vi "LOG_sim_2 (SubVI).vi"(3 "Data File":dbl[][](array[numeric]), 4 "Rotation":T5, 5 "Time":T3, 6 "TVA":T2, 7 "Position":T4, 9 "output Rocket Dynamics":T1) -> ()   [LabVIEW 2017]
panel:
  out "output array":dbl[](array[numeric])
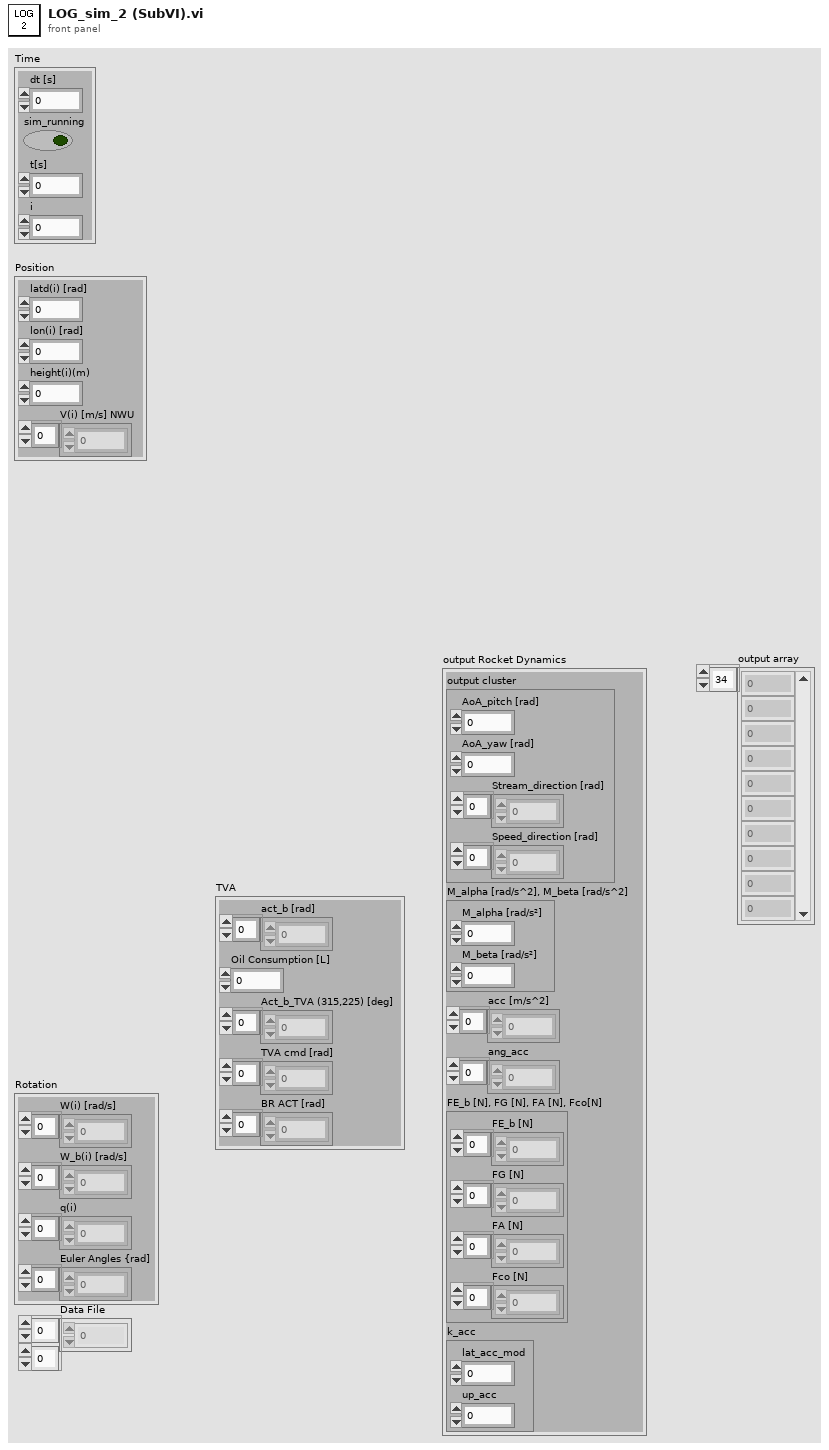
[diagram p1: front panel]
types:
  T1 = cluster{"output cluster":cluster{"AoA_pitch [rad]":dbl, "AoA_yaw [rad]":dbl, "Stream_direction [rad]":dbl[], "Speed_direction [rad]":dbl[]}, "M_alpha [rad/s^2], M_beta [rad/s^2]":cluster{"M_alpha [rad/s²]":dbl, "M_beta [rad/s²]":dbl}, "acc [m/s^2]":dbl[], "ang_acc":dbl[], "FE_b [N], FG [N], FA [N], Fco[N]":cluster{"FE_b [N]":dbl[], "FG [N]":dbl[], "FA [N]":dbl[], "Fco [N]":dbl[]}, "k_acc":cluster{"lat_acc_mod":dbl, "up_acc":dbl}}
  T2 = cluster{"act_b [rad]":dbl[], "Oil Consumption [L]":dbl, "Act_b_TVA (315,225) [deg]":dbl[], "TVA cmd [rad]":dbl[], "BR ACT [rad]":dbl[]}
  T3 = cluster{"dt [s]":dbl, "sim_running":bool, "t[s]":dbl, "i":i32}
  T4 = cluster{"latd(i) [rad]":dbl, "lon(i) [rad]":dbl, "height(i)(m)":dbl, "V(i) [m/s] NWU":dbl[]}
  T5 = cluster{"W(i) [rad/s]":dbl[], "W_b(i) [rad/s]":dbl[], "q(i)":dbl[], "Euler Angles {rad]":dbl[]}
  T6 = cluster{"M_alpha [rad/s²]":dbl, "M_beta [rad/s²]":dbl}
  T7 = cluster{"AoA_pitch [rad]":dbl, "AoA_yaw [rad]":dbl, "Stream_direction [rad]":dbl[], "Speed_direction [rad]":dbl[]}
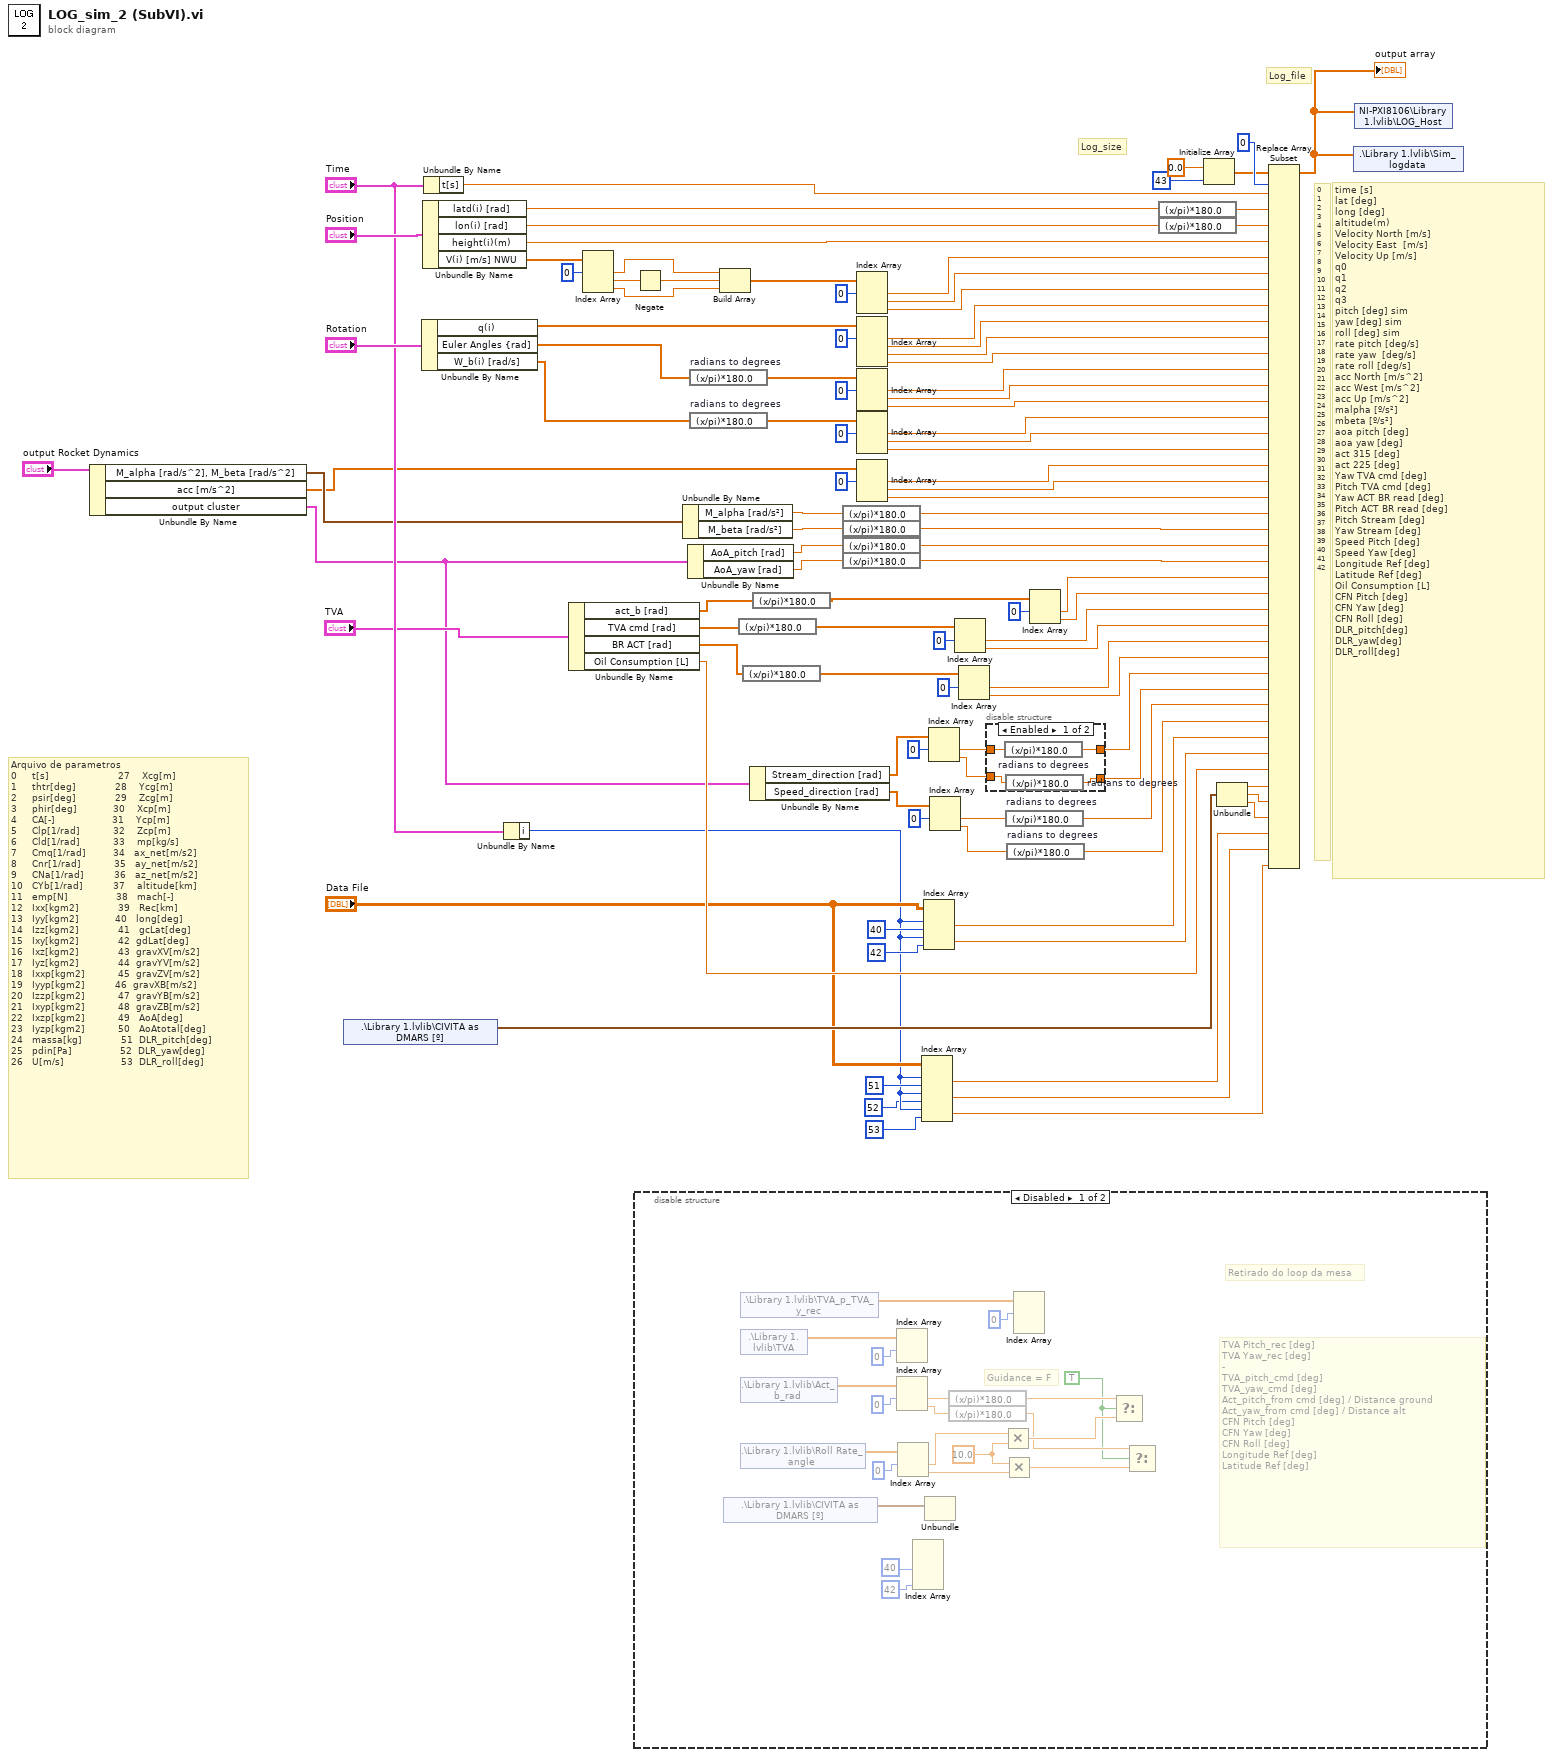
[diagram p0: block diagram]
diagram:
  # "Arquivo de parametros\n0     t[s]                       27    Xcg[m] \n1     thtr[deg]             28    Ycg[m]\n2     psir[deg]             29    Zcg[m]  \n3     phir[deg]            30    Xcp[m]       \n4     CA[-]                   31    Ycp[m]        \n5     Clp[1/rad]           32    Zcp[m]     \n6     Cld[1/rad]           33    mp[kg/s]        \n7     Cmq[1/rad]         34   ax_net[m/s2]         \n8     Cnr[1/rad]           35   ay_net[m/s2]      \n9     CNa[1/rad]          36   az_net[m/s2]      \n10   CYb[1/rad]          37    altitude[km]       \n11   emp[N]                38   mach[-]     \n12   Ixx[kgm2]             39   Rec[km]     \n13   Iyy[kgm2]            40   long[deg]     \n14   Izz[kgm2]             41   gcLat[deg]        \n15   Ixy[kgm2]             42  gdLat[deg]       \n16   Ixz[kgm2]             43  gravXV[m/s2]  \n17   Iyz[kgm2]             44  gravYV[m/s2]     \n18   Ixxp[kgm2]           45  gravZV[m/s2]         \n19   Iyyp[kgm2]          46  gravXB[m/s2]         \n20   Izzp[kgm2]           47  gravYB[m/s2]         \n21   Ixyp[kgm2]           48  gravZB[m/s2]           \n22   Ixzp[kgm2]           49   AoA[deg]             \n23   Iyzp[kgm2]           50   AoAtotal[deg]       \n24   massa[kg]             51  DLR_pitch[deg]    \n25   pdin[Pa]                52  DLR_yaw[deg]  \n26   U[m/s]                   53  DLR_roll[deg]"
  # "Log_file"
  # "Log_size"
  # "0\n1\n2\n3\n4\n5\n6\n7\n8\n9\n10\n11\n12\n13\n14\n15\n16\n17\n18\n19\n20\n21\n22\n23\n24\n25\n26\n27\n28\n29\n30\n31\n32\n33 34 35\n36373839\n40\n41\n42"
  # "time [s]\nlat [deg]\nlong [deg]\naltitude(m)\nVelocity North [m/s]\nVelocity East  [m/s]\nVelocity Up [m/s]\nq0\nq1\nq2\nq3\npitch [deg] sim\nyaw [deg] sim\nroll [deg] sim\nrate pitch [deg/s] \nrate yaw  [deg/s]\nrate roll [deg/s]\nacc North [m/s^2] \nacc West [m/s^2]\nacc Up [m/s^2]\nmalpha [º/s²]\nmbeta [º/s²]\naoa pitch [deg] \naoa yaw [deg]\nact 315 [deg] \nact 225 [deg]\nYaw TVA cmd [deg]\nPitch TVA cmd [deg]\nYaw ACT BR read [deg]\nPitch ACT BR read [deg]\nPitch Stream [deg]\nYaw Stream [deg]\nSpeed Pitch [deg]\nSpeed Yaw [deg]\nLongitude Ref [deg]\nLatitude Ref [deg]\nOil Consumption [L]\nCFN Pitch [deg]\nCFN Yaw [deg]\nCFN Roll [deg]\nDLR_pitch[deg]  \nDLR_yaw[deg] \nDLR_roll[deg]"
  n1 = Unbundle By Name("output Rocket Dynamics") -> ("M_alpha [rad/s^2], M_beta [rad/s^2]"=w11:T6, "acc [m/s^2]"=w10:dbl[], "output cluster"=w9:T7)
  n2 = shared-variable ".\\Library 1.lvlib\\CIVITA as DMARS [º]"() -> (w16:cluster{"phi":dbl, "theta":dbl, "psi":dbl})  [unwired: 1 in, 1 out]
  n3 = Unbundle By Name("Rotation") -> ("q(i)"=w103:dbl[], "Euler Angles {rad]"=w37:dbl[], "W_b(i) [rad/s]"=w36:dbl[])
  n4 = Unbundle By Name("Position") -> ("latd(i) [rad]"=w98:dbl, "lon(i) [rad]"=w99:dbl, "height(i)(m)"=w100:dbl, "V(i) [m/s] NWU"=w101:dbl[])
  n5 = Unbundle By Name("Time") -> ("t[s]"=w95:dbl)
  n6 = Unbundle By Name("Time") -> ("i"=w6:i32)
  n7 = Unbundle By Name("TVA") -> ("act_b [rad]"=w26:dbl[], "TVA cmd [rad]"=w28:dbl[], "BR ACT [rad]"=w21:dbl[], "Oil Consumption [L]"=w24:dbl)
  n8 = Index Array(array=w101, index #1=0 ("index")) -> (element #1=w73:dbl, element #2=w71:dbl, element #3=w74:dbl)  [unwired: 2 in]
  n9 = Negate(x=w71) -> (-x=w72:dbl)
  n10 = disable-structure shown="Disabled" {
    frame Disabled {
      w114 = TRUE ("s")
      w121 = 10.0 ("x")
      # "TVA Pitch_rec [deg]\nTVA Yaw_rec [deg]\n-\nTVA_pitch_cmd [deg]\nTVA_yaw_cmd [deg]\nAct_pitch_from cmd [deg] / Distance ground\nAct_yaw_from cmd [deg] / Distance alt\nCFN Pitch [deg]\nCFN Yaw [deg]\nCFN Roll [deg]\nLongitude Ref [deg]\nLatitude Ref [deg]"
      # "Retirado do loop da mesa"
      # "Guidance = F"
      n11 = shared-variable ".\\Library 1.lvlib\\CIVITA as DMARS [º]"() -> (w113:cluster{"phi":dbl, "theta":dbl, "psi":dbl})  [unwired: 1 in, 1 out]
      n12 = shared-variable ".\\Library 1.lvlib\\TVA_p_TVA_y_rec"() -> (w130:dbl[])  [unwired: 1 in, 1 out]
      n13 = shared-variable ".\\Library 1.lvlib\\TVA"() -> (w133:dbl[])  [unwired: 1 in, 1 out]
      n14 = shared-variable ".\\Library 1.lvlib\\Act_b_rad"() -> (w128:dbl[])  [unwired: 1 in, 1 out]
      n15 = shared-variable ".\\Library 1.lvlib\\Roll Rate_angle"() -> (w124:dbl[])  [unwired: 1 in, 1 out]
      n16 = Index Array(array=w133, index #1=0 ("index")) -> (element #1=w132:dbl, element #2=w131:dbl)  [unwired: 1 in]
      n17 = Index Array(array=w128, index #1=0 ("index")) -> (element #1=w127:dbl, element #2=w126:dbl)  [unwired: 1 in]
      n18 = Index Array(array=w124, index #1=0 ("index")) -> (element #1=w123:dbl, element #2=w122:dbl)  [unwired: 1 in]
      n19 = Index Array(index (col) #1=40 ("index"), index (row) #2=w108, index (col) #2=42 ("index")) -> (element #1=w106, index (row) #1=w108:i32, element #2=w105)  [unwired: 1 in]
      n20 = Unbundle(w113) -> ("phi"=w112:dbl, "theta"=w111:dbl, "psi"=w110:dbl)
      n21 = expression code="(x/pi)*180.0" ("radians to degrees")(w127) -> (w120:dbl)
      n22 = expression code="(x/pi)*180.0" ("radians to degrees")(w126) -> (w118:dbl)
      n23 = Multiply(x=w123, y=w121) -> (x*y=w119:dbl)
      n24 = Multiply(x=w121, y=w122) -> (x*y=w117:dbl)
      n25 = Index Array(array=w130, index #1=0 ("index")) -> (element #1=w137:dbl, element #2=w135:dbl, element #3=w136:dbl)  [unwired: 2 in]
      n26 = Select(t=w120, s=w114, f=w119) -> (s? t:f=w116:dbl)
      n27 = Select(t=w118, s=w114, f=w117) -> (s? t:f=w115:dbl)
    }
    frame Enabled {
    }
  }
  n28 = Unbundle By Name(w11) -> ("M_alpha [rad/s²]"=w87:dbl, "M_beta [rad/s²]"=w88:dbl)
  n29 = Unbundle By Name(w9) -> ("AoA_pitch [rad]"=w89:dbl, "AoA_yaw [rad]"=w90:dbl)
  n30 = expression code="(x/pi)*180.0" "radians to degrees"(w37) -> (w91:dbl[])
  n31 = expression code="(x/pi)*180.0" "radians to degrees"(w36) -> (w58:dbl[])
  n32 = Build Array(w73, w72, w74) -> (w104:dbl[])
  n33 = expression code="(x/pi)*180.0" ("radians to degrees")(w28) -> (w27:dbl[])
  n34 = expression code="(x/pi)*180.0" ("radians to degrees")(w21) -> (w23:dbl[])
  n35 = Unbundle By Name(w9) -> ("Stream_direction [rad]"=w92:dbl[], "Speed_direction [rad]"=w96:dbl[])
  n36 = expression code="(x/pi)*180.0" ("radians to degrees")(w26) -> (w25:dbl[])
  n37 = expression code="(x/pi)*180.0" ("radians to degrees")(w87) -> (w67:dbl)
  n38 = expression code="(x/pi)*180.0" ("radians to degrees")(w88) -> (w68:dbl)
  n39 = expression code="(x/pi)*180.0" ("radians to degrees")(w89) -> (w78:dbl)
  n40 = expression code="(x/pi)*180.0" ("radians to degrees")(w90) -> (w79:dbl)
  n41 = Index Array(array=w104, index #1=0 ("index")) -> (element #1=w46:dbl, element #2=w47:dbl, element #3=w48:dbl)  [unwired: 2 in]
  n42 = Index Array(array=w103, index #1=0 ("index")) -> (element #1=w50:dbl, element #2=w51:dbl, element #3=w52:dbl, element #4=w53:dbl)  [unwired: 3 in]
  n43 = Index Array(array=w91, index #1=0 ("index")) -> (element #1=w54:dbl, element #2=w55:dbl, element #3=w56:dbl)  [unwired: 2 in]
  n44 = Index Array(array=w58, index #1=0 ("index")) -> (element #1=w59:dbl, element #2=w60:dbl, element #3=w61:dbl)  [unwired: 2 in]
  n45 = Index Array(array=w10, index #1=0 ("index")) -> (element #1=w63:dbl, element #2=w64:dbl, element #3=w65:dbl)  [unwired: 2 in]
  n46 = Index Array(array="Data File", index (row) #1=w6, index (col) #1=51 ("index"), index (row) #2=w6, index (col) #2=52 ("index"), index (row) #3=w6, index (col) #3=53 ("index")) -> (element #1=w3:dbl, element #2=w2:dbl, element #3=w1:dbl)
  n47 = Index Array(array="Data File", index (row) #1=w6, index (col) #1=40 ("index"), index (row) #2=w6, index (col) #2=42 ("index")) -> (element #1=w32:dbl, element #2=w31:dbl)
  n48 = Index Array(array=w92, index #1=0 ("index")) -> (element #1=w75:dbl, element #2=w77:dbl)  [unwired: 1 in]
  n49 = Index Array(array=w96, index #1=0 ("index")) -> (element #1=w82:dbl, element #2=w80:dbl)  [unwired: 1 in]
  n50 = Index Array(array=w27, index #1=0 ("index")) -> (element #1=w85:dbl, element #2=w86:dbl)  [unwired: 1 in]
  n51 = Index Array(array=w23, index #1=0 ("index")) -> (element #1=w20:dbl, element #2=w17:dbl)  [unwired: 1 in]
  n52 = disable-structure shown="Enabled" {
    disable-tunnel: w75 -> [w142 w144]
    disable-tunnel: w77 -> [w141 w143]
    disable-tunnel: [w140 w144] -> w18
    disable-tunnel: [w139 w143] -> w19
    frame Enabled {
      n53 = expression code="(x/pi)*180.0" "radians to degrees"(w142) -> (w140:dbl)
      n54 = expression code="(x/pi)*180.0" "radians to degrees"(w141) -> (w139:dbl)
    }
    frame Disabled {
    }
  }
  n55 = expression code="(x/pi)*180.0" "radians to degrees"(w82) -> (w83:dbl)
  n56 = expression code="(x/pi)*180.0" "radians to degrees"(w80) -> (w84:dbl)
  n57 = Index Array(array=w25, index #1=0 ("index")) -> (element #1=w93:dbl, element #2=w94:dbl)  [unwired: 1 in]
  n58 = expression code="(x/pi)*180.0" ("radians to degrees")(w98) -> (w43:dbl)
  n59 = expression code="(x/pi)*180.0" ("radians to degrees")(w99) -> (w44:dbl)
  n60 = Initialize Array(0.0 ("element"), 43 ("dimension size")) -> (w40:dbl[])
  n61 = Unbundle(w16) -> ("phi"=w15:dbl, "theta"=w14:dbl, "psi"=w13:dbl)
  n62 = Replace Array Subset(array=w40, new element #1=w95, index #1=0 ("index"), new element #2=w43, new element #3=w44, new element #4=w100, new element #5=w46, new element #6=w47, new element #7=w48, new element #8=w50, new element #9=w51, new element #10=w52, new element #11=w53, new element #12=w54, new element #13=w55, new element #14=w56, new element #15=w59, new element #16=w60, new element #17=w61, new element #18=w63, new element #19=w64, new element #20=w65, new element #21=w67, new element #22=w68, new element #23=w78, new element #24=w79, new element #25=w93, new element #26=w94, new element #27=w85, new element #28=w86, new element #29=w20, new element #30=w17, new element #31=w18, new element #32=w19, new element #33=w83, new element #34=w84, new element #35=w32, new element #36=w31, new element #37=w24, new element #38=w15, new element #39=w14, new element #40=w13, new element #41=w3, new element #42=w2, new element #43=w1) -> (w30:dbl[])  [unwired: 42 in]
  "output array" <- w30
  n63 = shared-variable ".\\Library 1.lvlib\\Sim_logdata"(w30) -> ()  [unwired: 1 in, 1 out]
  n64 = shared-variable "NI-PXI8106\\Library 1.lvlib\\LOG_Host"(w30) -> ()  [unwired: 1 in, 1 out]
